vi "Move Control Position.vi"(7 "Sliding Speed (30)":u32=30, 8 "error in (no error)":errorcluster, 10 "Desired Position":T1, 11 "Obj Ref":refnum<vi>) -> (0 "error out":errorcluster, 1 "Old Position":T1, 2 "New Position":T1)   [LabVIEW 2018]
uses:
  <vilib>/Utility/miscctls.llb/LVPositionTypeDef.ctl
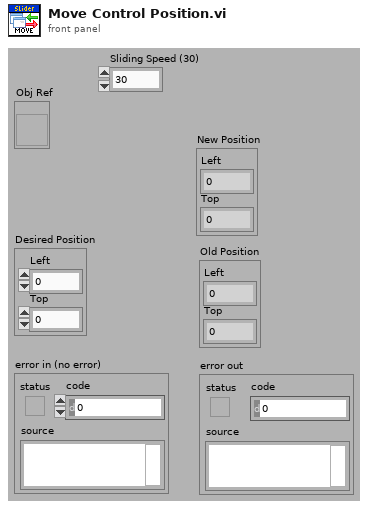
[diagram p1: front panel]
types:
  T1 = typedef "LVPositionTypeDef.ctl" = cluster{"Left":i32, "Top":i32}
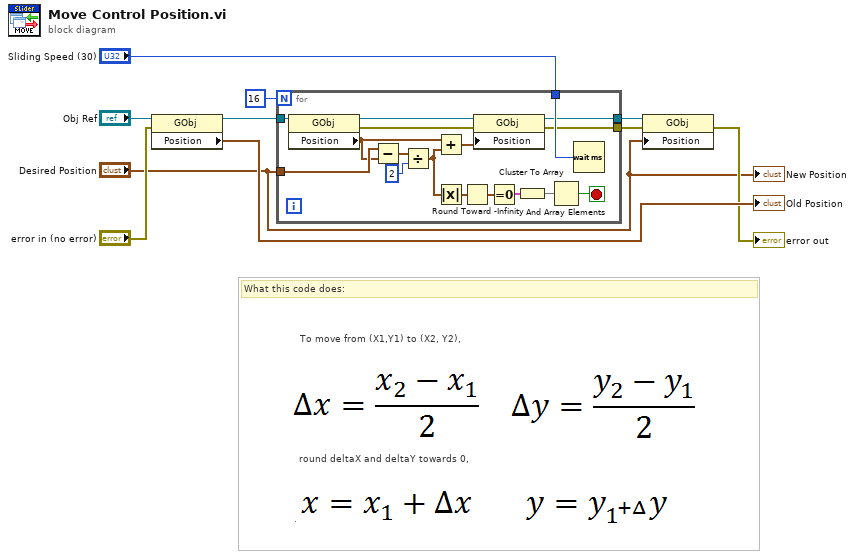
[diagram p0: block diagram]
diagram:
  # "round deltaX and deltaY towards 0,"
  # "To move from (X1,Y1) to (X2, Y2),"
  # "What this code does:"
  n1 = property on="Property Node" class="GObj"(reference="Obj Ref", error in="error in (no error)") -> (reference out=w8:refnum<vi>, "Position"=→"Old Position":T1)  [unwired: 1 out]
  n2 = for {
    N: 16 -> [_]
    tunnel: "Desired Position" -> [w27]
    tunnel: [w17] -> w3
    tunnel: "Sliding Speed (30)" -> [w18]
    tunnel: [w12] -> w5
    tunnel: w8 -> [w11]
    stop <- w19 stop-if-true
    n3 = property on="Property Node" class="GObj"(reference=w11) -> (reference out=w13:refnum<vi>, error out=w14:errorcluster, "Position"=w15:T1)  [unwired: 1 in]
    n4 = Subtract(x=w27, y=w15) -> (x-y=w26:T1)
    n5 = Divide(x=w26, y=2) -> (x/y=w22:cluster{"Left":dbl, "Top":dbl})
    n6 = Add(x=w15, y=w22) -> (x+y=w16:cluster{"Left":dbl, "Top":dbl})
    n7 = Absolute Value(x=w22) -> (abs(x)=w24:cluster{"Left":dbl, "Top":dbl})
    n8 = Round Toward -Infinity(1:w24) -> (0:w23:cluster{"Left":dbl, "Top":dbl})
    n9 = property on="Property Node" class="GObj"(reference=w13, error in=w14, "Position"=w16) -> (reference out=w12:refnum<vi>, error out=w17:errorcluster)
    n10 = Equal To 0?(x=w23) -> (x = 0?=w21:cluster{"Left":bool, "Top":bool})
    n11 = Cluster To Array(cluster=w21) -> (array=w20:bool[])
    n12 = And Array Elements(Boolean array=w20) -> (logical AND=w19:bool)
    n13 = Wait (ms)(milliseconds to wait=w18) -> ()  [unwired: 1 out]
  }
  n14 = property on="Property Node" class="GObj"(reference=w5, error in=w3, "Position"="Desired Position") -> (error out=→"error out":errorcluster)  [unwired: 1 out]
  "New Position" <- "Desired Position"
